vi "LCD_Setting_UI.vi"(6 "Analysis_Setting IN":T1 {"Analysis_Type" items=["None", "PatternMatch", "Edge Detection", "Barcode 1D", "Barcode 2D", "Clamp", "Clamp MAX", "Particle", "Histogram", "Straight Edge", "Circle", "Shape Detect", "OCR", "Contour", "ColorMatch"]}, 8 "error in (no error)":errorcluster, 9 "ProjectName":string, 10 "ROI List IN":refnum<vi>, 11 "Vision_Image":T6(plugin-control)) -> (0 "error out":errorcluster, 1 "Cancel?":bool, 3 "Analysis_Setting":T1 {"Analysis_Type" items=["None", "PatternMatch", "Edge Detection", "Barcode 1D", "Barcode 2D", "Clamp", "Clamp MAX", "Particle", "Histogram", "Straight Edge", "Circle", "Shape Detect", "OCR", "Contour", "ColorMatch"]})   [LabVIEW 2015]
uses:
  Controls/Analysis_Setting.ctl
  Controls/Analysis_Type.ctl
  Controls/_UI Command Cluster/LCD_UI Command Cluster.ctl
  <vilib>/userdefined/High Color/IMAQdx.ctl
  Controls/LCD/Analysis_LCD_Parameter.ctl
  <vilib>/vision/NI_Vision_Development_Module.lvlib
panel:
  out "Numeric":i32
  in  "Done":bool
  in  "LCD_UI Command":T3(ring)
  in  "Cancel":bool
  in  "LCDTab":T4(tab)
  in  "Number of Matches Requested":i32=1 min=1 max=9999
  in  "Snap?":bool
  in  "Simulaation":bool
  in  "ROI":T5
  out "Output value":dbl
  out "ROI Out":T5
  # "27"
  # "270"
  # "147"
  # "55"
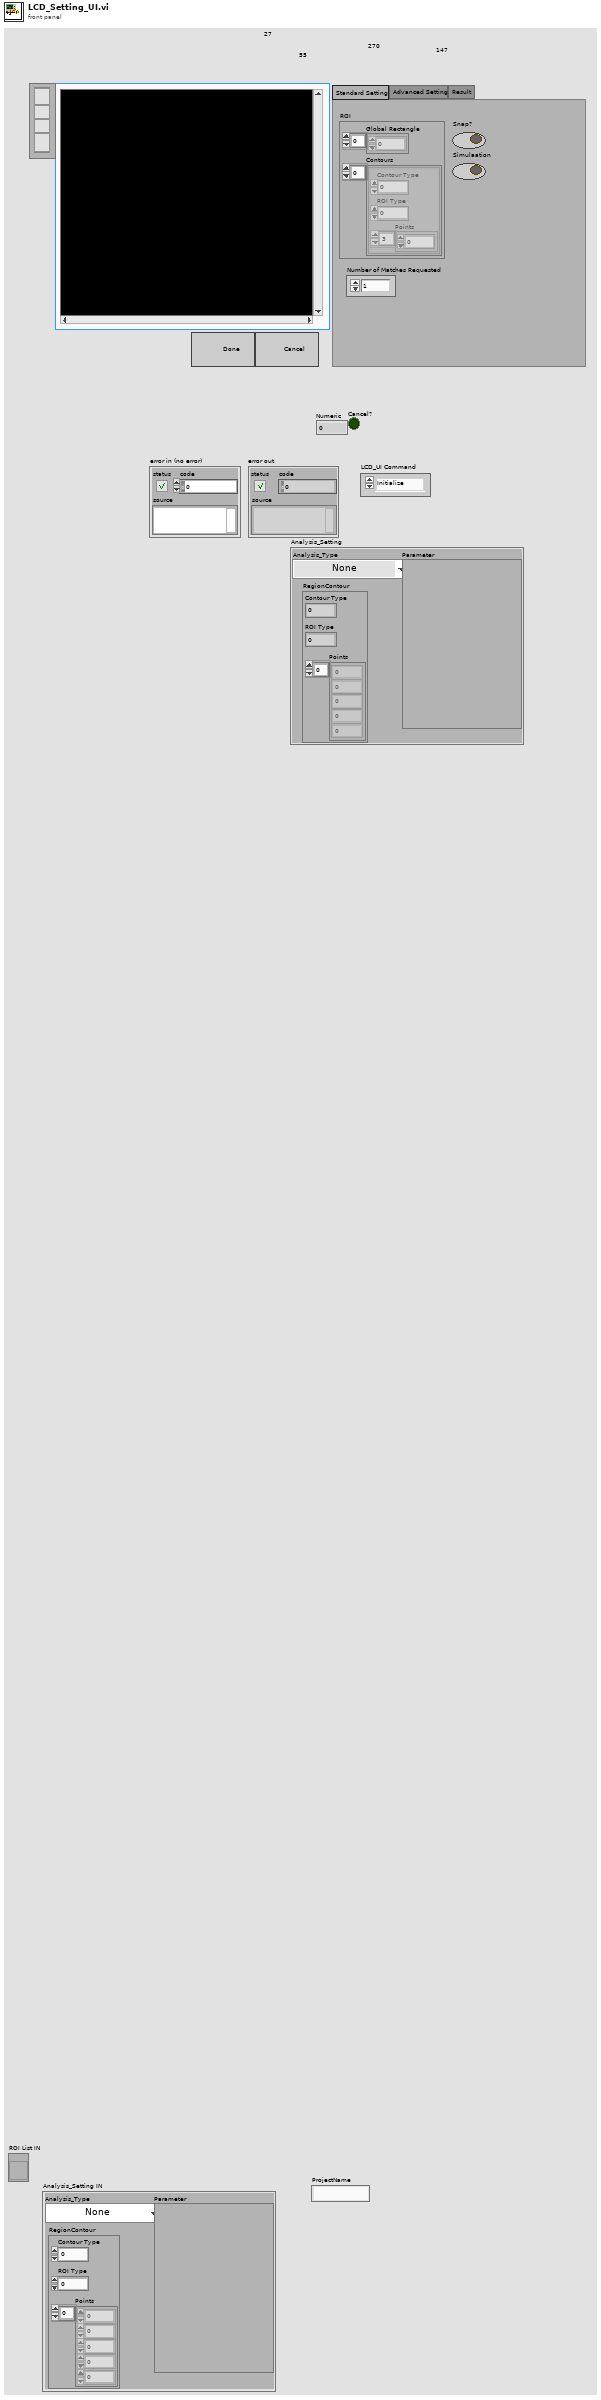
[diagram p1: front panel]
types:
  T1 = typedef "Analysis_Setting.ctl" = cluster{"Analysis_Type":T2, "RegionContour":cluster{"Contour Type":u32, "ROI Type":u32, "Points":i32[]}, "Parameter":variant}
  T2 = typedef "Analysis_Type.ctl" = u16
  T3 = enum16{"Initialize", "Done", "Run Algorithm", "Cancel"}
  T4 = enum32{"Standard Setting", "Advanced Setting", "Result"}
  T5 = cluster{"Global Rectangle":i32[], "Contours":cluster{"Contour Type":u32, "ROI Type":u32, "Points":i32[]}[]}
  T6 = typedef "IMAQ Image.ctl" = refnum<image>
  T7 = typedef "LCD_UI Command Cluster.ctl" = cluster{"LCD_UI Command":enum16{"Initialize", "Done", "Run Algorithm", "Cancel"}, "ROI":cluster{"Global Rectangle":i32[], "Contours":cluster{"Contour Type":u32, "ROI Type":u32, "Points":i32[]}[]}, "Number of Matches Requested":i32, "Snap Simulation Mouse Down":bool}
  T8 = typedef "IMAQ Line" = cluster{"Start X":i32, "Start Y":i32, "End X":i32, "End Y":i32}
  T9 = typedef "IMAQdx.ctl" = refnum<k21>
  T10 = cluster{"Contour Type":u32, "ROI Type":u32, "Points":i32[]}
  T11 = typedef "Analysis_LCD_Parameter.ctl" = cluster{"ROI":cluster{"Global Rectangle":i32[], "Contours":cluster{"Contour Type":u32, "ROI Type":u32, "Points":i32[]}[]}, "Number of Matches Requested":i32}
  T12 = typedef "ROI Descriptor" = cluster{"Global Rectangle":i32[], "Contours":cluster{"ID":enum32{"External", "Internal"}, "Type":u32, "Coordinates":i32[]}[]}
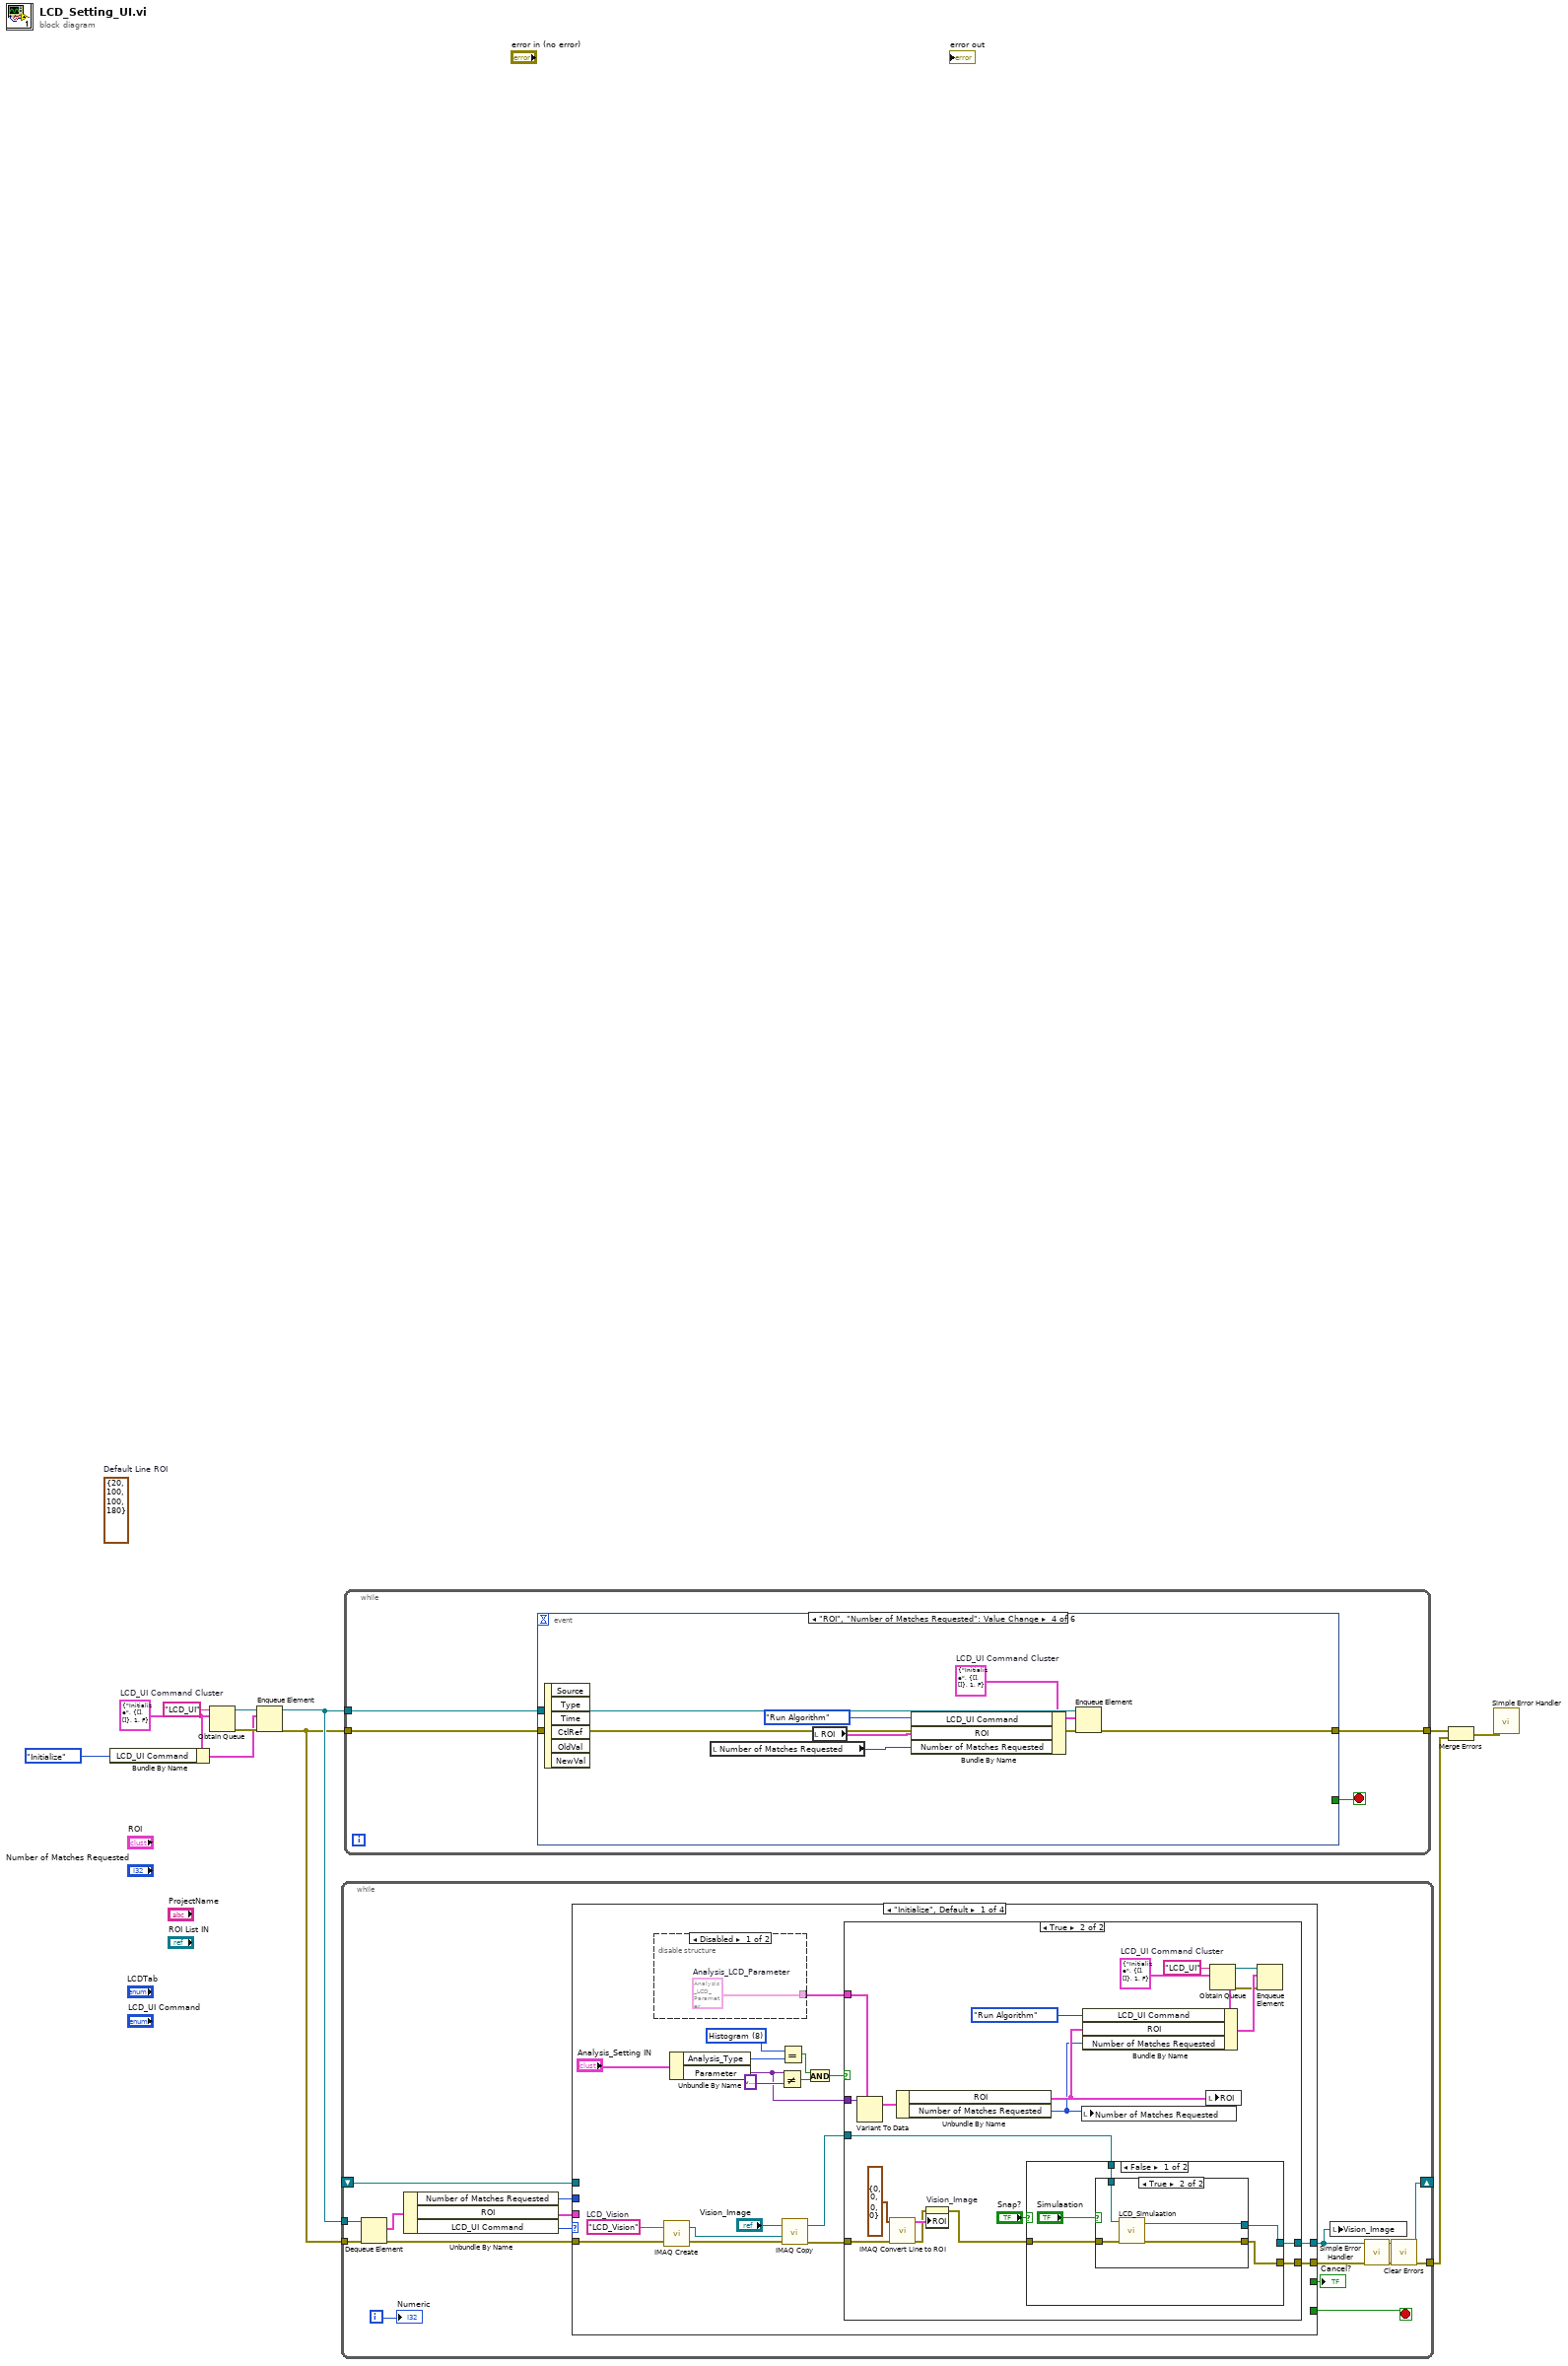
[diagram p0: block diagram]
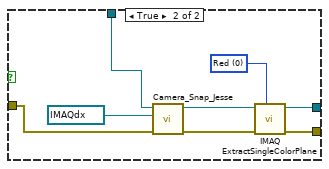
[diagram p5: hidden frame]
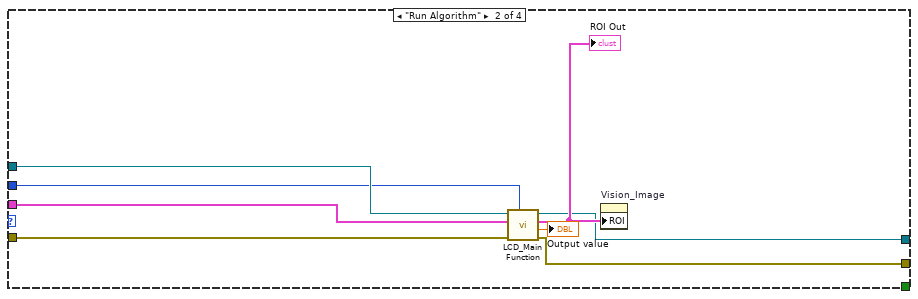
[diagram p6: hidden frame]
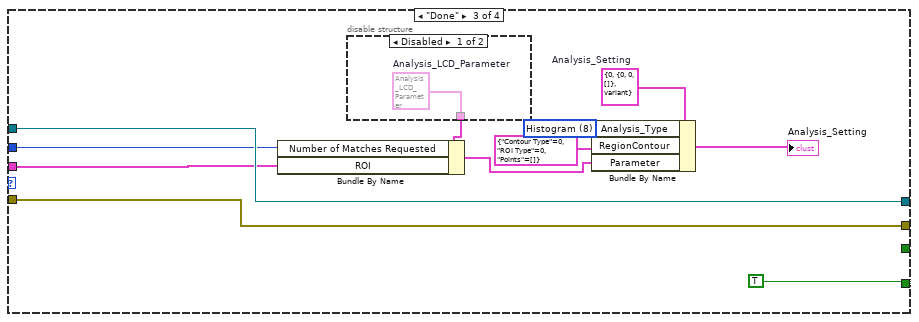
[diagram p7: hidden frame]
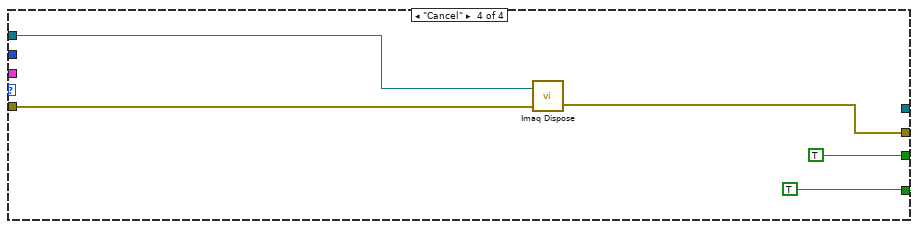
[diagram p9: hidden frame]
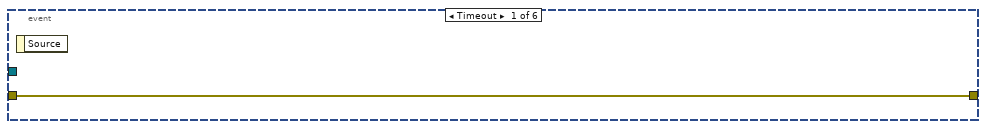
[diagram p10: hidden frame]
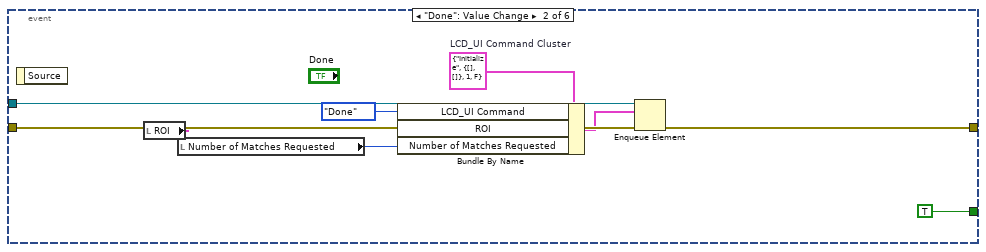
[diagram p11: hidden frame]
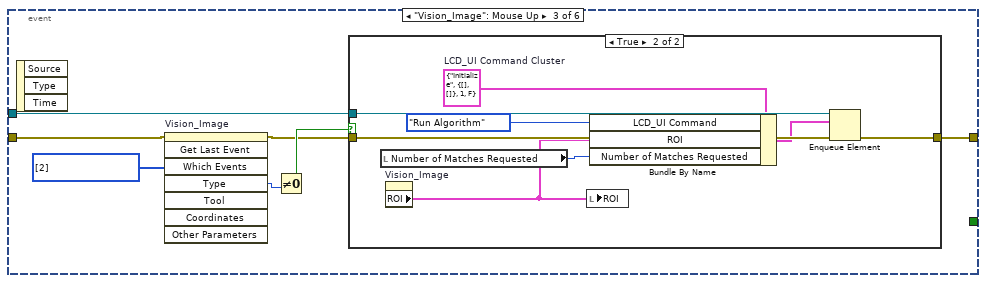
[diagram p12: hidden frame]
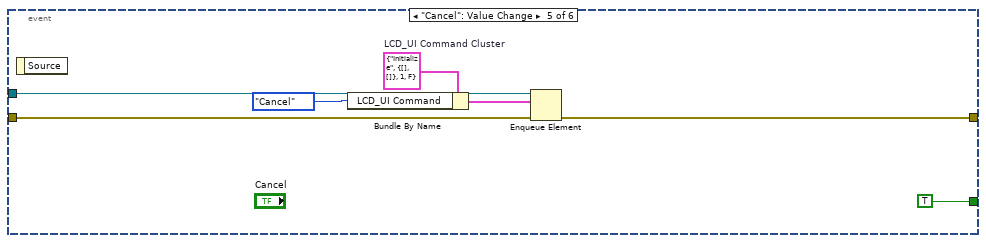
[diagram p14: hidden frame]
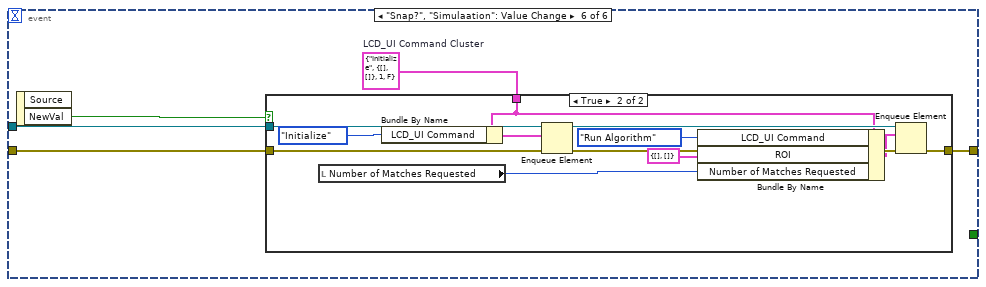
[diagram p15: hidden frame]
diagram:
  w3 = T7 {"LCD_UI Command"=enum."Initialize", "ROI"={"Global Rectangle"=[], "Contours"=[]}, "Number of Matches Requested"=1, "Snap Simulation Mouse Down"=FALSE}  # LCD_UI Command Cluster
  (unwired) T8 {"Start X"=20, "Start Y"=100, "End X"=100, "End Y"=180}  # Default Line ROI
  n1 = Bundle By Name(cluster=w3, "LCD_UI Command"=T3."Initialize" ("Barcode 1D_UI Command")) -> (w4:T7)
  n2 = Obtain Queue(name (unnamed)="LCD_UI", element data type=w3) -> (queue out=w11:refnum<queue>, error out=w10:errorcluster)  [unwired: 3 in, 1 out]
  n3 = Enqueue Element(queue=w11, element=w4, error in (no error)=w10) -> (queue out=w2:refnum<queue>, error out=w1:errorcluster)  [unwired: 1 in, 1 out]
  n4 = while {
    tunnel: w2 -> [w26]
    tunnel: w1 -> [w25]
    shift-right: [w14] -> _
    shift-left: _ -> [w20]
    tunnel: [w12] -> w7
    i -> [w19]
    stop <- w21 stop-if-true
    n5 = Dequeue Element(queue=w26, error in (no error)=w25) -> (element=w22:T7, error out=w23:errorcluster)  [unwired: 1 in, 2 out]
    n6 = Unbundle By Name(w22) -> ("Number of Matches Requested"=w15:i32, "ROI"=w16:T5, "LCD_UI Command"=w24:T3)
    n7 = case shown="\"Initialize\", Default" w24 {
      tunnel: w23 -> [w34 w94 w103 w109]
      tunnel: [w44 w92 w103 w108] -> w18
      tunnel: [_ _ TRUE TRUE] -> w21
      tunnel: [w43 w87 w104 _] -> w14
      tunnel: w20 -> [_ w93 w104 w110]
      tunnel: [_ _ _ TRUE] -> w17
      tunnel: w16 -> [_ w90 w96 _]
      tunnel: w15 -> [_ w88 w95 _]
      frame "Initialize", Default {
        w35 = "LCD_Vision"  # LCD_Vision
        w40 = T2 8 items=["None", "PatternMatch", "Edge Detection", "Barcode 1D", "Barcode 2D", "Clamp", "Clamp MAX", "Particle", "Histogram", "Straight Edge", "Circle", "Shape Detect", "OCR", "Contour", "ColorMatch"] ("x")
        n8 = disable-structure shown="Disabled" {
          disable-tunnel: [w45 _] -> w27
          frame Disabled {
            w45 = T11 {"ROI"={"Global Rectangle"=[27, 55, 270, 147], "Contours"=[{"Contour Type"=0, "ROI Type"=3, "Points"=[27, 55, 270, 147]}]}, "Number of Matches Requested"=1}  # Analysis_LCD_Parameter
          }
          frame Enabled {
          }
        }
        n9 = call "IMAQ Create"("Image Name"=w35, "error in (no error)"=w34) -> ("New Image"=w32:T6, "error out"=w31:errorcluster)  [unwired: 3 in]
        n10 = Unbundle By Name("Analysis_Setting IN") -> ("Analysis_Type"=w39:T2, "Parameter"=w28:variant)
        n11 = Not Equal?(x=w28, y=variant) -> (x != y?=w41:bool)
        n12 = Equal?(x=w40, y=w39) -> (x = y?=w42:bool)
        n13 = call "IMAQ Copy"("error in (no error)"=w31, "Image Dst"=w32, "Image Src"="Vision_Image") -> ("error out"=w30:errorcluster, "Image Dst Out"=w29:T6)  [unwired: 3 in]
        n14 = And(x=w42, y=w41) -> (x .and. y?=w36:bool)
        n15 = case shown="True" w36 {
          tunnel: w30 -> [w46 w59]
          tunnel: [w46 w57] -> w44
          tunnel: [w47 w58] -> w43
          tunnel: w29 -> [w47 w60]
          tunnel: w28 -> [_ w67]
          tunnel: w27 -> [_ w56]
          frame False {
          }
          frame True {
            w55 = T7 {"LCD_UI Command"=enum."Initialize", "ROI"={"Global Rectangle"=[], "Contours"=[]}, "Number of Matches Requested"=1, "Snap Simulation Mouse Down"=FALSE}  # LCD_UI Command Cluster
            n16 = Variant To Data(type=w56, Variant=w67) -> (data=w66:T11)  [unwired: 1 in, 1 out]
            n17 = call "IMAQ Convert Line to ROI"("error in (no error)"=w59, "Line"=T8 {"Start X"=0, "Start Y"=0, "End X"=0, "End Y"=0}) -> ("error out"=w62:errorcluster, "ROI Descriptor"=w63:T12)  [unwired: 7 in]
            n18 = Unbundle By Name(w66) -> ("ROI"=w49:T5, "Number of Matches Requested"=w48:i32)
            n19 = property on="Vision_Image" class="ImageControl"(error in=w62, "ROI"=w63) -> (error out=w61:errorcluster)  [unwired: 1 in, 1 out]
            n20 = case shown="False" "Snap?" {
              tunnel: [w72 w82] -> w57
              tunnel: [w71 w81] -> w58
              tunnel: w61 -> [w70 w79]
              tunnel: w60 -> [w68 w80]
              frame False {
                n21 = case shown="True" "Simulaation" {
                  tunnel: [w73 w77] -> w72
                  tunnel: [w74 w76] -> w71
                  tunnel: w70 -> [w73 w78]
                  tunnel: w68 -> [w74 w75]
                  frame False {
                  }
                  frame True {
                    n22 = call "LCD_Simulaation.vi"("error in (no error)"=w78, "Refnum in"=w75) -> ("error out"=w77:errorcluster, "Refnum out"=w76:T6)  [unwired: 8 in]
                  }
                }
              }
              frame True {
                w84 = 0 items=["Red", "Green", "Blue", "Hue", "Saturation", "Luminance", "Value", "Intensity"] ("Color Plane")
                n23 = call "Camera_Snap_Jesse.vi"("error in (no error)"=w79, "Camera Session In"=T9 "cam0", "Image In"=w80) -> ("error out"=w83:errorcluster, "New Image"=w85:T6)  [unwired: 7 in]
                n24 = call "IMAQ ExtractSingleColorPlane"("Color Plane"=w84, "error in (no error)"=w83, "Image Src"=w85) -> ("error out"=w82:errorcluster, "Image Dst Out"=w81:T6)  [unwired: 1 in, 6 out]
              }
            }
            n25 = local write "Number of Matches Requested"(w48) -> ()
            n26 = Bundle By Name(cluster=w55, "LCD_UI Command"=T3."Run Algorithm" ("Barcode 1D_UI Command"), "ROI"=w49, "Number of Matches Requested"=w48) -> (w54:T7)
            n27 = local write "ROI"(w49) -> ()
            n28 = Obtain Queue(name (unnamed)="LCD_UI", element data type=w55) -> (queue out=w50:refnum<queue>, error out=w51:errorcluster)  [unwired: 3 in, 1 out]
            n29 = Enqueue Element(queue=w50, element=w54, error in (no error)=w51) -> ()  [unwired: 1 in, 3 out]
          }
        }
      }
      frame "Run Algorithm" {
        n30 = call "LCD_Main Function.vi"("Number of Matches Requested"=w88, "error in (no error)"=w94, "ROI Descriptor"=w90, "Refnum in"=w93) -> ("error out"=w92:errorcluster, "Output value"=→"Output value":dbl, "ROI"=w89:T5, "Refnum out"=w87:T6)  [unwired: 4 in]
        "ROI Out" <- w89
        n31 = property on="Vision_Image" class="ImageControl"("ROI"=w89) -> ()  [unwired: 2 in, 2 out]
      }
      frame "Done" {
        w101 = T2 8 items=["None", "PatternMatch", "Edge Detection", "Barcode 1D", "Barcode 2D", "Clamp", "Clamp MAX", "Particle", "Histogram", "Straight Edge", "Circle", "Shape Detect", "OCR", "Contour", "ColorMatch"] ("Analysis_Type")
        w102 = T1 {"Analysis_Type"=0, "RegionContour"={"Contour Type"=0, "ROI Type"=0, "Points"=[]}, "Parameter"=variant}  # Analysis_Setting
        n32 = disable-structure shown="Disabled" {
          disable-tunnel: [w106 _] -> w99
          frame Disabled {
            w106 = T11 {"ROI"={"Global Rectangle"=[27, 55, 270, 147], "Contours"=[{"Contour Type"=0, "ROI Type"=3, "Points"=[27, 55, 270, 147]}]}, "Number of Matches Requested"=1}  # Analysis_LCD_Parameter
          }
          frame Enabled {
          }
        }
        n33 = Bundle By Name(cluster=w99, "Number of Matches Requested"=w95, "ROI"=w96) -> (w98:T11)
        n34 = Bundle By Name(cluster=w102, "Analysis_Type"=w101, "RegionContour"=T10 {"Contour Type"=0, "ROI Type"=0, "Points"=[]}, "Parameter"=w98) -> (→"Analysis_Setting":T1)
      }
      frame "Cancel" {
        n35 = call "Imaq Dispose"("Image"=w110, "error in (no error)"=w109) -> ("error out"=w108:errorcluster)  [unwired: 4 in]
      }
    }
    "Cancel?" <- w17
    n36 = local write "Vision_Image"(w14) -> ()
    n37 = call <vilib>:"Simple Error Handler.vi"("error in (no error)"=w18) -> ("error out"=w13:errorcluster)  [unwired: 4 in, 4 out]
    n38 = call <vilib>:"Clear Errors.vi"("error in (no error)"=w13) -> ("error out"=w12:errorcluster)  [unwired: 5 in, 1 out]
    "Numeric" <- w19
  }
  n39 = while {
    tunnel: w2 -> [w115]
    tunnel: w1 -> [w114]
    tunnel: [w112] -> w8
    stop <- w113 stop-if-true
    n40 = event shown="[3] \"ROI\", \"Number of Matches Requested\": Value Change" {
      selector: _ -> [_ _ _ _ _ _]
      dyn-events: _ -> [_ _ _ _ _ _]
      timeout: _ -> [_ _ _ _ _ _]
      tunnel: w115 -> [_ w125 w132 w149 w156 w161]
      tunnel: w114 -> [w116 w124 w129 w148 w155 w160]
      tunnel: [_ TRUE _ _ TRUE _] -> w113
      tunnel: [w116 w123 w126 w147 w153 w158] -> w112
      event Timeout {
        n41 = event-data() -> ()  [unwired: 1 in, 1 out]
      }
      event "Done": Value Change {
        w122 = T7 {"LCD_UI Command"=enum."Initialize", "ROI"={"Global Rectangle"=[], "Contours"=[]}, "Number of Matches Requested"=1, "Snap Simulation Mouse Down"=FALSE}  # LCD_UI Command Cluster
        n42 = event-data() -> ()  [unwired: 1 in, 1 out]
        n43 = local read "ROI"() -> (w117:T5)
        n44 = local read "Number of Matches Requested"() -> (w118:i32)
        n45 = Bundle By Name(cluster=w122, "LCD_UI Command"=T3."Done" ("Edge Detection_UI Command"), "ROI"=w117, "Number of Matches Requested"=w118) -> (w120:T7)
        n46 = Enqueue Element(queue=w125, element=w120, error in (no error)=w124) -> (error out=w123:errorcluster)  [unwired: 1 in, 2 out]
      }
      event "Vision_Image": Mouse Up {
        w130 = i32[] [2] items=["No Event"=0, "Click Event"=1, "Draw Event"=2, "Size Event"=4, "Scroll Event"=5, "Double Click Event"=8] ("Which Events")
        n47 = event-data() -> ()  [unwired: 1 in, 3 out]
        n48 = invoke on="Vision_Image" class="ImageControl" method="Get Last Event"(error in=w129, "Which Events"=w130) -> (error out=w128:errorcluster, "Type"=w127:i32)  [unwired: 6 in, 6 out]
        n49 = Not Equal To 0?(x=w127) -> (x != 0?=w131:bool)
        n50 = case shown="True" w131 {
          tunnel: w132 -> [_ w141]
          tunnel: w128 -> [w133 w140]
          tunnel: [w133 w136] -> w126
          frame False {
          }
          frame True {
            w139 = T7 {"LCD_UI Command"=enum."Initialize", "ROI"={"Global Rectangle"=[], "Contours"=[]}, "Number of Matches Requested"=1, "Snap Simulation Mouse Down"=FALSE}  # LCD_UI Command Cluster
            n51 = local read "Number of Matches Requested"() -> (w135:i32)
            n52 = property on="Vision_Image" class="ImageControl"() -> ("ROI"=w134:T5)  [unwired: 2 in, 2 out]
            n53 = local write "ROI"(w134) -> ()
            n54 = Bundle By Name(cluster=w139, "LCD_UI Command"=T3."Run Algorithm", "ROI"=w134, "Number of Matches Requested"=w135) -> (w137:T7)
            n55 = Enqueue Element(queue=w141, element=w137, error in (no error)=w140) -> (error out=w136:errorcluster)  [unwired: 1 in, 2 out]
          }
        }
      }
      event "ROI", "Number of Matches Requested": Value Change {
        w146 = T7 {"LCD_UI Command"=enum."Initialize", "ROI"={"Global Rectangle"=[], "Contours"=[]}, "Number of Matches Requested"=1, "Snap Simulation Mouse Down"=FALSE}  # LCD_UI Command Cluster
        n56 = event-data() -> ()  [unwired: 1 in, 6 out]
        n57 = local read "Number of Matches Requested"() -> (w142:i32)
        n58 = local read "ROI"() -> (w143:T5)
        n59 = Bundle By Name(cluster=w146, "LCD_UI Command"=T3."Run Algorithm" ("Barcode 1D_UI Command"), "ROI"=w143, "Number of Matches Requested"=w142) -> (w144:T7)
        n60 = Enqueue Element(queue=w149, element=w144, error in (no error)=w148) -> (error out=w147:errorcluster)  [unwired: 1 in, 2 out]
      }
      event "Cancel": Value Change {
        w152 = T7 {"LCD_UI Command"=enum."Initialize", "ROI"={"Global Rectangle"=[], "Contours"=[]}, "Number of Matches Requested"=1, "Snap Simulation Mouse Down"=FALSE}  # LCD_UI Command Cluster
        n61 = event-data() -> ()  [unwired: 1 in, 1 out]
        n62 = Bundle By Name(cluster=w152, "LCD_UI Command"=T3."Cancel" ("Barcode 1D_UI Command")) -> (w151:T7)
        n63 = Enqueue Element(queue=w156, element=w151, error in (no error)=w155) -> (error out=w153:errorcluster)  [unwired: 1 in, 2 out]
      }
      event "Snap?", "Simulaation": Value Change {
        w157 = T7 {"LCD_UI Command"=enum."Initialize", "ROI"={"Global Rectangle"=[], "Contours"=[]}, "Number of Matches Requested"=1, "Snap Simulation Mouse Down"=FALSE}  # LCD_UI Command Cluster
        n64 = event-data() -> ("NewVal"=w159:bool)  [unwired: 1 in, 1 out]
        n65 = case shown="True" w159 {
          tunnel: w161 -> [_ w174]
          tunnel: w160 -> [w162 w173]
          tunnel: w157 -> [_ w169]
          tunnel: [w162 w167] -> w158
          frame False {
          }
          frame True {
            n66 = local read "Number of Matches Requested"() -> (w163:i32)
            n67 = Bundle By Name(cluster=w169, "LCD_UI Command"=T3."Initialize" ("Barcode 1D_UI Command")) -> (w172:T7)
            n68 = Enqueue Element(queue=w174, element=w172, error in (no error)=w173) -> (queue out=w171:refnum<queue>, error out=w170:errorcluster)  [unwired: 1 in, 1 out]
            n69 = Bundle By Name(cluster=w169, "LCD_UI Command"=T3."Run Algorithm" ("Barcode 1D_UI Command"), "ROI"=T5 {"Global Rectangle"=[], "Contours"=[]}, "Number of Matches Requested"=w163) -> (w168:T7)
            n70 = Enqueue Element(queue=w171, element=w168, error in (no error)=w170) -> (error out=w167:errorcluster)  [unwired: 1 in, 2 out]
          }
        }
      }
    }
  }
  n71 = Merge Errors(w8, w7) -> (w6:errorcluster)
  n72 = call <vilib>:"Simple Error Handler.vi"("error in (no error)"=w6) -> ()  [unwired: 4 in, 5 out]
